vi "F5xxx_pq_set_mode.vi"(8 "error in":errorcluster, 10 "mode":enum16{"OFF", "CH", "DAMPL"}(ring), 11 "VISA in":refnum<visa-resource-name>) -> (0 "error out":errorcluster, 3 "VISA out":refnum<visa-resource-name>)   [LabVIEW 2013]
uses:
  Fluke 5XXX Series Multicalibrators.lvlib
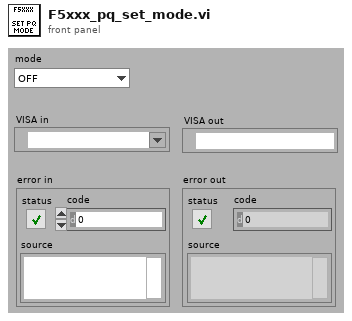
[diagram p1: front panel]
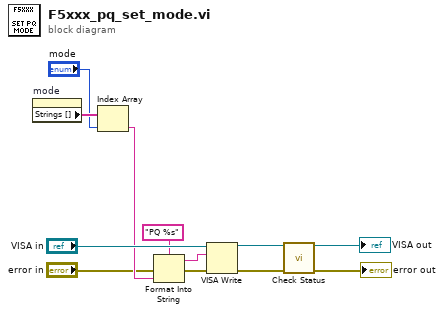
[diagram p0: block diagram]
diagram:
  n1 = property on="mode" class="Enum (strict)"() -> ("Strings []"=w9:string[])  [unwired: 2 in, 2 out]
  n2 = Index Array(array=w9, index="mode") -> (element=w7:string)
  n3 = Format Into String(format string="PQ %s", error in="error in", w7) -> (resulting string=w11:string, error out=w6:errorcluster)  [unwired: 1 in]
  n4 = VISA Write(VISA resource name="VISA in", write buffer=w11, error in (no error)=w6) -> (VISA resource name out=w3:refnum<visa-resource-name>, error out=w4:errorcluster)  [unwired: 1 out]
  n5 = call "Check Status.vi"("VISA resource name"=w3, "error in (no error)"=w4) -> ("VISA resource name out"=→"VISA out":refnum<visa-resource-name>, "error out"=→"error out":errorcluster)  [unwired: 12 in]
